vi "Find Instr.vi"(8 "error in":errorcluster, 11 "Instrument array":refnum<class "Instrument.lvclass">[](array[class])) -> (0 "error out":errorcluster, 1 "All Ready?":bool, 2 "Status array":T1(array[cluster]), 3 "Instrument array out":refnum<class "Instrument.lvclass">[](array[class]))   [LabVIEW 2012]
uses:
  LabVIEW-programs/Instruments/Utility Classes/Instrument/Instrument.lvclass
panel:
  out "busybar":bool[](array[boolean])
  out "done?":bool
  # "Find Instruments"
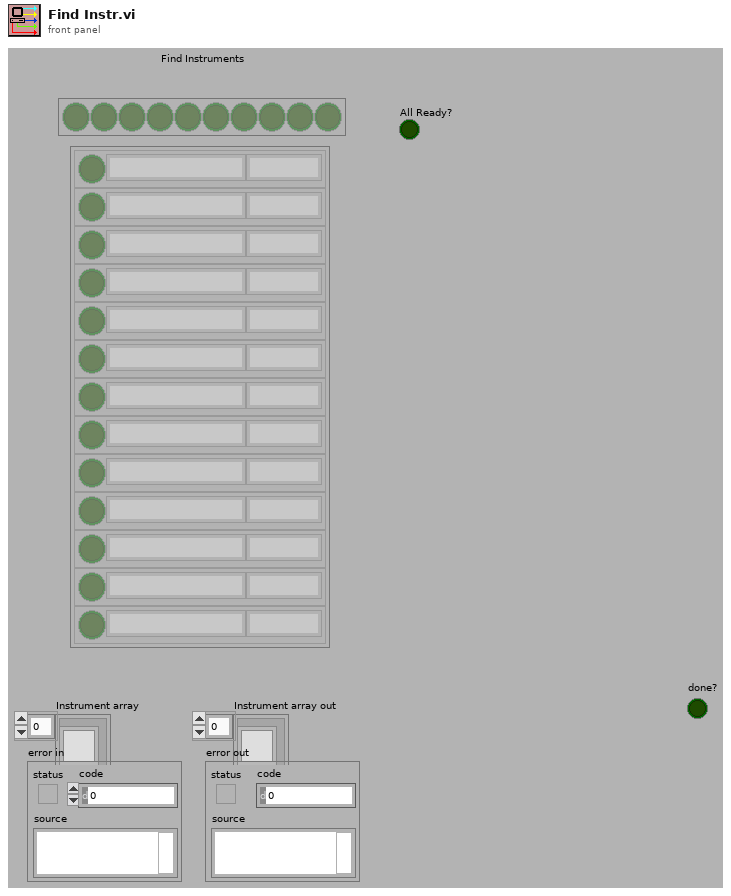
[diagram p1: front panel]
types:
  T1 = cluster{"On?":bool, "Name":string, "Status":string}[]
  T2 = cluster{"Ready?":bool, "Name":string, "Status":string}
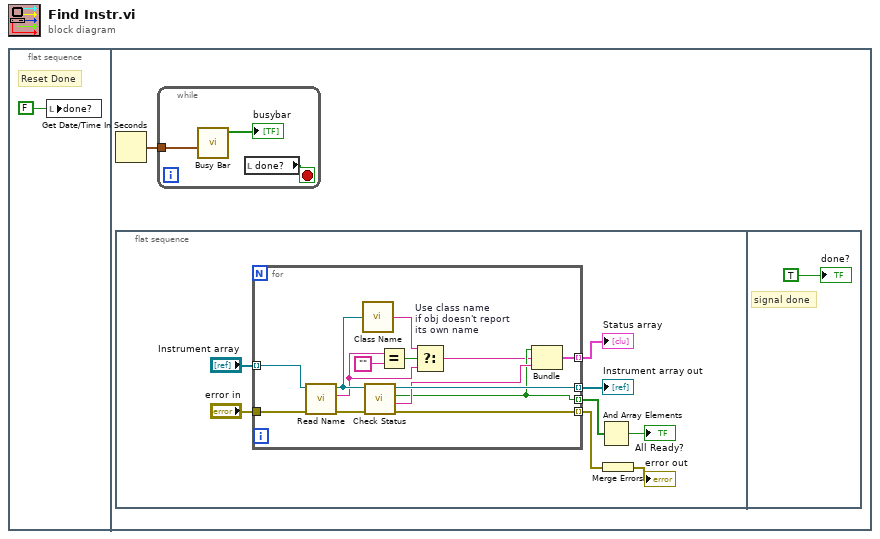
[diagram p0: block diagram]
diagram:
  n1 = flat-sequence {
    frame #0 {
      # "Reset Done"
      n2 = local write "done?"(FALSE) -> ()
    }
    frame #1 {
      n3 = Get Date/Time In Seconds() -> (seconds since 1Jan1904=w2:timestamp)
      n4 = flat-sequence {
        frame #0 {
          n5 = for {
            tunnel: "Instrument array" -> [w20] mode=indexing
            tunnel: [w23] -> w9 mode=indexing
            tunnel: [w18] -> w7 mode=indexing
            tunnel: "error in" -> [w22]
            tunnel: [w21] -> w5 mode=indexing
            tunnel: [w17] -> w3 mode=indexing
            n6 = call-dynamic "Read Name.vi"("error in (no error)"=w22, "Instrument.lvclass in"=w20) -> ("error out"=w24:errorcluster, "Name"=w12:string, "Instrument.lvclass out"=w16:refnum<class "Instrument.lvclass">)  [unwired: 7 out]
            n7 = call "Class Name.vi"("LabVIEW Object"=w16) -> ("Classname"=w14:string)
            n8 = call-dynamic "Check Status.vi"("error in (no error)"=w24, "Instrument in"=w16) -> ("error out"=w21:errorcluster, "Status"=w19:string, "Ready?"=w18:bool, "Instrument out"=w23:refnum<class "Instrument.lvclass">)  [unwired: 6 out]
            n9 = Equal?(x=w12, y="") -> (x = y?=w13:bool)
            n10 = Select "Use class name\nif obj doesn't report\nits own name"(t=w14, s=w13, f=w12) -> (s? t:f=w11:string)
            n11 = Bundle("Ready?"=w18, "Name"=w11, "Status"=w19) -> (w17:T2)  [unwired: 1 out]
          }
          "Instrument array out" <- w9
          "Status array" <- w3
          n12 = And Array Elements(Boolean array=w7) -> (logical AND=→"All Ready?":bool)
          n13 = Merge Errors(w5) -> (→"error out":errorcluster)
        }
        frame #1 {
          # "signal done"
          "done?" <- TRUE
        }
      }
      n14 = while {
        tunnel: w2 -> [w26]
        stop <- w28 stop-if-true
        n15 = call "Busy Bar.vi"("basetime"=w26) -> ("Busy Bar"=→"busybar":bool[])  [unwired: 2 in, 8 out]
        n16 = local read "done?"() -> (w28:bool)
      }
    }
  }
